vi "DIO Block Write Bank.vi"(10 "DO.DMA_CNTR":u16, 11 "DMA FIFO IN":refnum<k21>="DO") -> (0 "DO.DMA_IDL":bool, 2 "FIFO OUT":fxp<+,20,20>)   [LabVIEW 2021]
uses:
  <vilib>/rvi/DataTransferAndStorage/Container/XNode/niFpgaContainer.xnode
  <vilib>/rvi/FIFO/Fifo_Resource/niFpgaFifoEmulationRefIn.vi
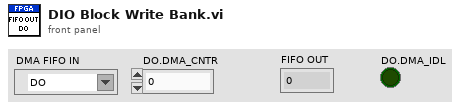
[diagram p1: front panel]
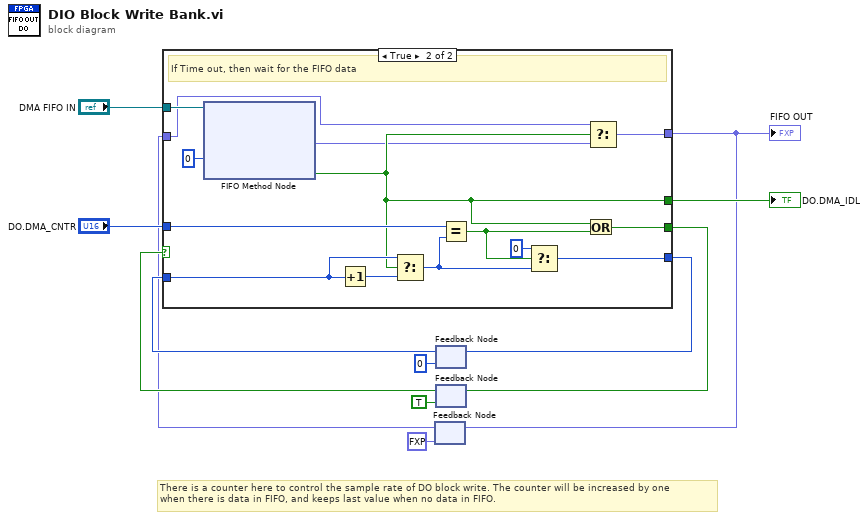
[diagram p0: block diagram]
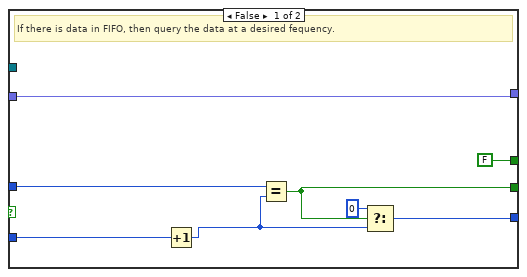
[diagram p2: hidden frame]
diagram:
  # "There is a counter here to control the sample rate of DO block write. The counter will be increased by one \nwhen there is data in FIFO, and keeps last value when no data in FIFO."
  n1 = feedback #1(fxp<+,20,20> 0.0 ("t")) -> (w2:fxp<+,20,20>)
  n2 = feedback #2(u16 0 ("t")) -> (w5:u16)
  n3 = feedback #3(TRUE ("Timed Out?")) -> (w10:bool)
  n4 = case shown="True" w10 {
    tunnel: [w14 w21] -> w1
    tunnel: "DO.DMA_CNTR" -> [w18 w28]
    tunnel: [w15 w33] -> w11
    tunnel: [FALSE ("Timed Out?") w24] -> w4
    tunnel: "DMA FIFO IN" -> [_ w25]
    tunnel: [w16 w27] -> w6
    tunnel: w5 -> [w17 w26]
    tunnel: w2 -> [w14 w22]
    frame False {
      # "If there is data in FIFO, then query the data at a desired fequency."
      n5 = Increment(x=w17) -> (x+1=w13:u16)
      n6 = Equal?(x=w18, y=w13) -> (x = y?=w15:bool)
      n7 = Select(t=u16 0, s=w15, f=w13) -> (s? t:f=w16:u16)
    }
    frame True {
      # "If Time out, then wait for the FIFO data"
      n8 = xnode ("FIFO Method Node")("Timeout"=0, "FIFO In"=w25) -> ("Element"=w23:fxp<+,20,20>, "Timed Out?"=w24:bool)  [unwired: 1 out]
      n9 = Increment(x=w26) -> (x+1=w32:u16)
      n10 = Select(t=w26, s=w24, f=w32) -> (s? t:f=w30:u16)
      n11 = Equal?(x=w28, y=w30) -> (x = y?=w29:bool)
      n12 = Select(t=u16 0, s=w29, f=w30) -> (s? t:f=w27:u16)
      n13 = Or(x=w24, y=w29) -> (x .or. y?=w33:bool)
      n14 = Select(t=w22, s=w24, f=w23) -> (s? t:f=w21:fxp<+,20,20>)
    }
  }
  "DO.DMA_IDL" <- w4
  "FIFO OUT" <- w1
  n15 = feedback-in #1(w1) -> ()
  n16 = feedback-in #2(w6) -> ()
  n17 = feedback-in #3(w11) -> ()
